vi "Write Data.vi"(7 "IP":i16, 8 "error in (no error)":errorcluster, 9 "Port":T1, 10 "Instructions":refnum<k21>, 11 "MPU in":refnum<class "MPU.lvclass">) -> (0 "error out":errorcluster, 2 "Numeric":i16, 3 "MPU out":refnum<class "MPU.lvclass">)   [LabVIEW 2018, in "Modbus_Processing_Unit.lvlib" / "MPU.lvclass"]
uses:
  MPU.lvclass
  PortType.ctl
  MPU.lvclass/MPU.ctl
  <vilib>/rvi/DataTransferAndStorage/Container/Common/niFpgaContainerExecOnDevCompGetState.vi
  <vilib>/rvi/Emulation/niFpgaEmulationIsFPGAContextNoSignature.vi
  <vilib>/rvi/DataTransferAndStorage/Container/Common/niFpgaContainerGetUniqueNameForEmu.vi
  <vilib>/rvi/Emulation/niFpgaProcessEmulError.vi
  <vilib>/rvi/Emulation/niFpgaSctlEmulationGetInTimedLoop.vi
  <vilib>/rvi/errors/nirviReportUnexpectedCaseInternalError (U32).vi
  <vilib>/rvi/Memory/Memory_Emulation/niFpgaMemoryEmulationCacheClearOnFirstRun.vi
  <vilib>/rvi/Memory/Memory_Emulation/nirvimemoryEmulationManagerCache_MakeExclusive.vi
  <vilib>/rvi/Memory/Memory_Emulation/niFpgaMemoryEmulationValidateCache.vi
  <vilib>/rvi/Memory/Memory_Emulation/nirvimemoryEmulationManagerCache_InsertValue.vi
  <vilib>/Utility/error.llb/Clear Errors.vi
  <vilib>/rvi/Memory/Memory_Emulation/nirvimemoryEmulationManagerCache_ReleaseExclusive.vi
  <vilib>/rvi/Memory/Memory_Emulation/nirvimemoryEmulationManagerCache_GetValue.vi
  <vilib>/rvi/Memory/Memory_Emulation/nirvimemoryEmulationManagerCache_SetValue.vi
  <vilib>/rvi/Emulation/niFpgaSctlEmulationResourceMgr.vi
  <vilib>/rvi/Emulation/niFpgaGetClockAttributes.vi
  <vilib>/rvi/Emulation/niFpgaEmulationReportErrorSimple.vi
  <vilib>/rvi/Emulation/niFpgaCriticalErrorInLSC.vi
  <vilib>/rvi/DataTransferAndStorage/Container/XNode/niFpgaContainer.xnode
  <vilib>/rvi/Memory/Memory_Emulation/niFpgaMemoryEmulationRefIn.vi
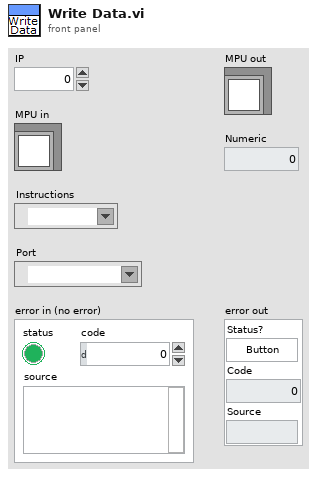
[diagram p1: front panel]
types:
  T1 = typedef "PortType.ctl" = refnum<k21>
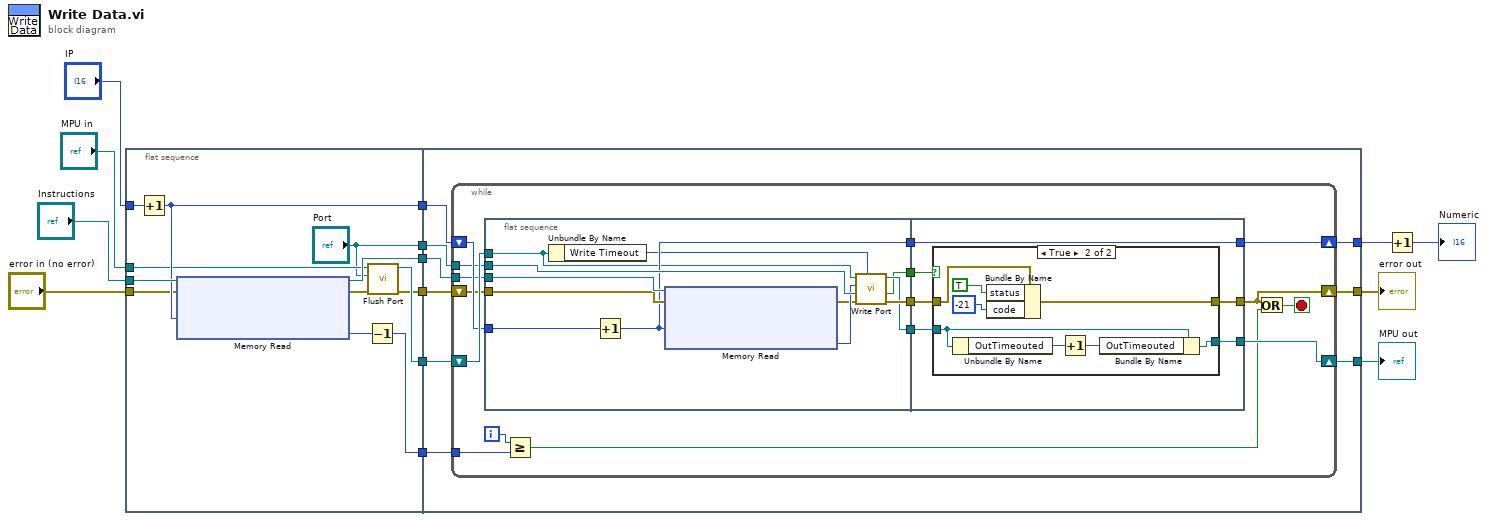
[diagram p0: block diagram]
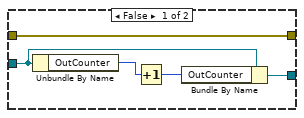
[diagram p2: hidden frame]
diagram:
  n1 = flat-sequence {
    tunnel: "MPU in" -> [w19]
    tunnel: "IP" -> [w26]
    tunnel: "Instructions" -> [w25]
    tunnel: "error in (no error)" -> [w20]
    tunnel: [w23] -> w6
    tunnel: [w18] -> w5
    tunnel: [w24] -> w4
    tunnel: [w22] -> w3
    tunnel: ["Port"] -> w2
    tunnel: [w16] -> w1
    tunnel: [w35] -> w14
    tunnel: [w34] -> w13
    tunnel: [w33] -> w12
    tunnel: w6 -> [w32]
    tunnel: w5 -> [w31]
    tunnel: w4 -> [w30]
    tunnel: w3 -> [w29]
    tunnel: w2 -> [w28]
    tunnel: w1 -> [w27]
    frame #0 {
      n2 = Increment(x=w26) -> (x+1=w23:i16)
      n3 = xnode ("Memory Read")("Address"=w23, "error in (no error)"=w20, "Memory In"=w25) -> ("Data"=w21:u8, "error out"=w17:errorcluster, "Memory Out"=w24:refnum<k21>)
      n4 = Decrement(x=w21) -> (x-1=w22:u8)
      n5 = call-dynamic "Flush Port.vi"("error in (no error)"=w17, "Port"="Port", "MPU in"=w19) -> ("error out"=w16:errorcluster, "MPU out"=w18:refnum<class "MPU.lvclass">)  [unwired: 7 in]
    }
    frame #1 {
      n6 = while {
        tunnel: w28 -> [w49]
        shift-right: [w47] -> w33
        shift-left: w32 -> [w50]
        shift-right: [w40] -> w34
        shift-left: w27 -> [w48]
        shift-right: [w46] -> w35
        shift-left: w31 -> [w51]
        tunnel: w30 -> [w37]
        tunnel: w29 -> [w36]
        i -> [w39]
        stop <- w41 stop-if-true
        n7 = flat-sequence {
          tunnel: w51 -> [w53]
          tunnel: w50 -> [w63]
          tunnel: w49 -> [w62]
          tunnel: w37 -> [w61]
          tunnel: w48 -> [w59]
          tunnel: [w57] -> w45
          tunnel: [w56] -> w44
          tunnel: [w55] -> w43
          tunnel: [w54] -> w42
          tunnel: [w67] -> w46
          tunnel: [w69] -> w47
          tunnel: w45 -> [w69]
          tunnel: w44 -> [w65]
          tunnel: w43 -> [w68]
          tunnel: w42 -> [w66]
          tunnel: [w64] -> w40
          frame #0 {
            n8 = Unbundle By Name(w53) -> ("Write Timeout"=w52:u16)
            n9 = Increment(x=w63) -> (x+1=w57:i16)
            n10 = xnode ("Memory Read")("Address"=w57, "error in (no error)"=w59, "Memory In"=w61) -> ("Data"=w60:u8, "error out"=w58:errorcluster)  [unwired: 1 out]
            n11 = call-dynamic "Write Port.vi"("Timeout"=w52, "error in (no error)"=w58, "Port"=w62, "Data"=w60, "MPU in"=w53) -> ("error out"=w56:errorcluster, "Timeouted"=w54:bool, "MPU out"=w55:refnum<class "MPU.lvclass">)  [unwired: 4 in]
          }
          frame #1 {
            n12 = case shown="True" w66 {
              tunnel: w68 -> [w74 w82]
              tunnel: [w73 w81] -> w67
              tunnel: w65 -> [w70 w78]
              tunnel: [w70 w77] -> w64
              frame False {
                n13 = Unbundle By Name(w74) -> ("OutCounter"=w72:u64)
                n14 = Increment(x=w72) -> (x+1=w71:u64)
                n15 = Bundle By Name(cluster=w74, "OutCounter"=w71) -> (w73:refnum<class "MPU.lvclass">)
              }
              frame True {
                n16 = Unbundle By Name(w82) -> ("OutTimeouted"=w80:u64)
                n17 = Bundle By Name(cluster=w78, "status"=TRUE, "code"=-21) -> (w77:errorcluster)
                n18 = Increment(x=w80) -> (x+1=w79:u64)
                n19 = Bundle By Name(cluster=w82, "OutTimeouted"=w79) -> (w81:refnum<class "MPU.lvclass">)
              }
            }
          }
        }
        n20 = Greater Or Equal?(x=w39, y=w36) -> (x >= y?=w38:bool)
        n21 = Or(x=w40, y=w38) -> (x .or. y?=w41:bool)
      }
    }
  }
  n22 = Increment(x=w12) -> (x+1=→"Numeric":i16)
  "MPU out" <- w14
  "error out" <- w13
